vi "Set System Image.vi"   [LabVIEW 2017, in "nisyscfg.lvlib"]
doc: "Applies a system image file or folder—a copy of the contents and software on a primary hard drive of a system. Applying the image to the system restores it to the state captured on the image."
uses:
  <vilib>/nisyscfg/nisyscfg.lvlib
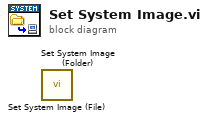
[diagram p0: block diagram]
diagram:
  n1 = call <vilib>:"Set System Image (File).vi"() -> ()  [unwired: 10 in, 2 out]
  n2 = call <vilib>:"Set System Image (Folder).vi"() -> ()  [unwired: 10 in, 2 out]
